vi "Set_VI_Ref.vi"(8 "error in (no error)":errorcluster, 11 "Class 1 in":refnum<class "Class 1.lvclass">) -> (0 "error out":errorcluster, 2 "Core_Reference_VI out":refnum<vi>, 3 "Class 1 out":refnum<class "Class 1.lvclass">)   [LabVIEW 2021, in "Class 1.lvclass"]
uses:
  Class 1.lvclass
  Files_Module/Modules/Sample_Panel_1.vi
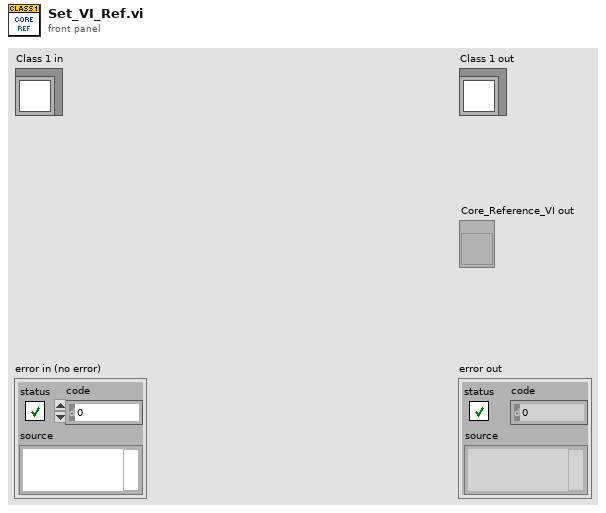
[diagram p1: front panel]
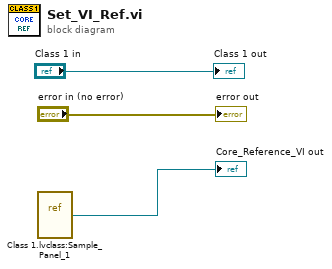
[diagram p0: block diagram]
diagram:
  n1 = vi-ref "Class 1.lvclass:Sample_Panel_1.vi"() -> (→"Core_Reference_VI out":refnum<vi>)
  "error out" <- "error in (no error)"
  "Class 1 out" <- "Class 1 in"
